vi "SystemTime_GetTime.vi"(8 "Fehler (Eingang, kein Fehler)":errorcluster caption="Error_In", 11 "OXYGEN Ref In":refnum<visa-resource-name>) -> (0 "Fehler (Ausgang)":errorcluster caption="Error_Out", 1 "communication_data":T1, 2 "System Time":string, 3 "OXYGEN Ref Out":refnum<visa-resource-name>)   [LabVIEW 2020, in "OXYGEN_Datastream.lvlib"]
doc: "Queries the system time."
uses:
  OXYGEN_Datastream.lvlib
  TypeDefs/Cluster_RawCommData.ctl
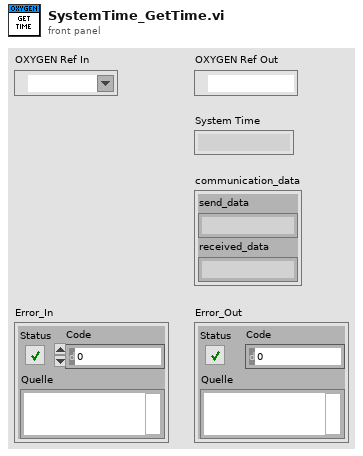
[diagram p1: front panel]
types:
  T1 = typedef "OXYGEN_Datastream.lvlib/Cluster_RawCommData.ctl" = cluster{"send_data":string, "received_data":string}
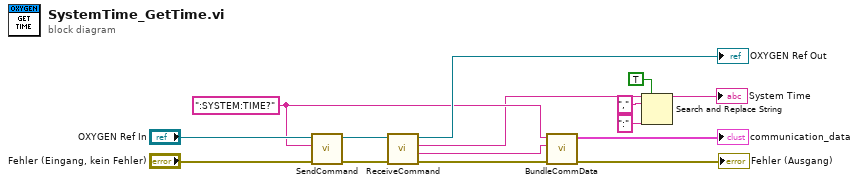
[diagram p0: block diagram]
diagram:
  w10 = ":SYSTEM:TIME?" ("Schreibpuffer")
  n1 = call "SendCommand.vi"("error in (no error)"="Fehler (Eingang, kein Fehler)", "String to Send"=w10, "OXY_SCPI Reseource In"="OXYGEN Ref In") -> ("error out"=w12:errorcluster, "OXY_SCPI Reseource Out"=w11:refnum<visa-resource-name>)  [unwired: 7 in]
  n2 = call "ReceiveCommand.vi"("error in (no error)"=w12, "OXY_SCPI Reseource In"=w11) -> ("error out"=w8:errorcluster, "received Data with Header"=w1:string, "received Data"=w6:string, "OXY_SCPI Reseource Out"=→"OXYGEN Ref Out":refnum<visa-resource-name>)  [unwired: 6 in]
  n3 = call "BundleCommData.vi"("error in (no error)"=w8, "received_data"=w1, "send_data"=w10) -> ("error out"=→"Fehler (Ausgang)":errorcluster, "communication_data"=→"communication_data":T1)  [unwired: 7 in]
  n4 = Search and Replace String(replace all?=TRUE ("replace all? (F)"), input string=w6, search string=",", replace string=":" ("replace string (\"\")")) -> (result string=→"System Time":string)  [unwired: 4 in, 3 out]
